vi "SwissSPAD Live_Save SS3 Data to HDF5_DVI.vi"(4 "Compression Level (0-9)":u8=9 max=9, 6 "Compression":bool, 7 "10-bit Gate Image":bool, 8 "error in (no error)":errorcluster, 9 "File Path::n":string="SS2 Live Gate Data Q", 10 "Gate Names":string[](array[string]), 11 "HDF5 ref":T1 format="%.0x") -> (0 "error out":errorcluster)   [LabVIEW 2021]
uses:
  <vilib>/addons/h5labview2/base/hid_t.ctl
  SwissSPAD Live_Settings List.ctl
  SwissSPAD Live_SS3 DAQ Parameters.ctl
  SwissSPAD Live_SS3 Gate Definition.ctl
  SS3 Gate Width Definition Mode.ctl
  SwissSPAD Live_Gate Type.ctl
  <vilib>/Utility/error.llb/DialogType.ctl
  <vilib>/addons/h5labview2/file/H5F.lvlib
  <vilib>/addons/h5labview2/group/H5G.lvlib
  Notebook/Notebook.lvlib
  Rich Text Box/Rich Text Box.lvlib
  Variant/Variant to Data/Variant to Data.lvlib
panel:
  out "File Path":string
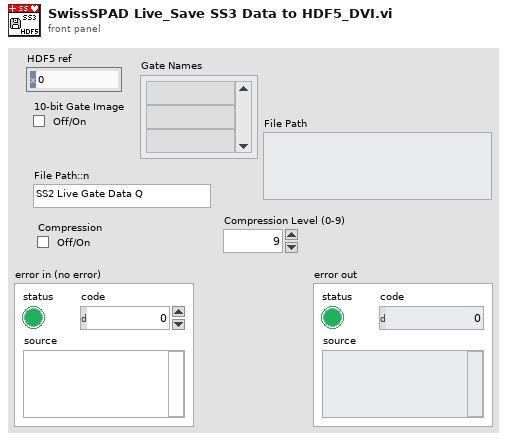
[diagram p1: front panel]
types:
  T1 = typedef "hid_t.ctl" = i32
  T2 = typedef "SwissSPAD Live_Settings List.ctl" = enum16{"FPGA:Bottom Half", "FPGA:Top Half", "FPGA:Bottom Bitfile Path", "FPGA:Top Bitfile Path", "FPGA:Bottom Bitstream Version", "FPGA:Top Bitstream Version", "FPGA:Auto Reset FPGA", "FPGA:Bottom FPGA Serial Number", "FPGA:Top FPGA Serial Number", "FPGA:Detector PCB Version", "Acquisition Parameters:Microlens", "Acquisition Parameters:SS2 DAQ Parameters", "Acquisition Parameters:Gate Configuration Array", "Acquisition Parameters:SS3 DAQ Parameters", "Acquisition Parameters:Buffer Size (# 8-bit Gates)", "File Information:File Information", "File Information:# Datasets in Series", "File Information:Scrambled File Flag", "File Information:SS3 Gate Slip Correction", "File Information:SS3 Hot Pixel Mismatch Detection", "File Information:Delay between Datasets", "File Information:Save Sum of All Gates Preview", "Image Parameters:Image ROI Information", "Image Parameters:Image Binning Options", "Image Parameters:SS3 Displayed Image", "Image Parameters:Image Display Options", "Image Parameters:Use Histogram Cursors", "Image Parameter:FPGA Data to Display", "UI Settings:Histogram Bins Number", "UI Settings:Histogram Bin Size", "UI Settings:Use Image Display Options", "UI Settings:Verbose Settings", "UI Settings:Verbose Saving"}
  T3 = typedef "SwissSPAD Live_Gate Type.ctl" = enum16{"INT", "G2"}
  T4 = typedef "SwissSPAD Live_SS3 DAQ Parameters.ctl" = cluster{"10 bits":bool, "# Exposure Sequences":u32, "# 1-bit Frame per Gate":u32, "Gate Shift":u32, "# Gate Pairs per Set":u32, "# Sets":u32, "Laser Period":dbl[unit], "Sync Period":dbl[unit], "Gate Offset":u32, "Auto-adjust Gate Offset":bool, "Gate Definition":T5, "Gate Width (ns)":dbl, "Reversed Shift":bool, "Intensity Mode":bool, "Gate Definition Mode":T6}
  T5 = typedef "SwissSPAD Live_SS3 Gate Definition.ctl" = cluster{"gs_psincdec_0":u32, "gs_psincdec_1":u32, "gs_no_shift_adj_1":u32, "gate_adj_2":u32}
  T6 = typedef "SS3 Gate Width Definition Mode.ctl" = enum32{"Item 0", "Item 1"}
  T7 = typedef "DialogType.ctl" = u16
  T8 = typedef "SwissSPAD Live_File Saving Task Information.ctl" = cluster{"File Path::n":string, "# Saved Images":i32, "# Images (Total)":i32, "File Size (Bytes)":i64}
  T9 = typedef "Rich Text Box.lvlib/Text Formatting.ctl" = cluster{"Font":string, "Text Color":T10, "Text Background Color":T10, "Text Style":enum16{"Regular", "Bold", "Italic", "Underline", "Strikeout"}, "Font Size (Points)":dbl, "Text Alignment":i32}
  T10 = typedef "Rich Text Box.lvlib/Text Colors.ctl" = enum16{"Unchanged", "Black", "Blue", "Brown", "Gray", "Green", "Orange", "Pink", "Red", "White"}
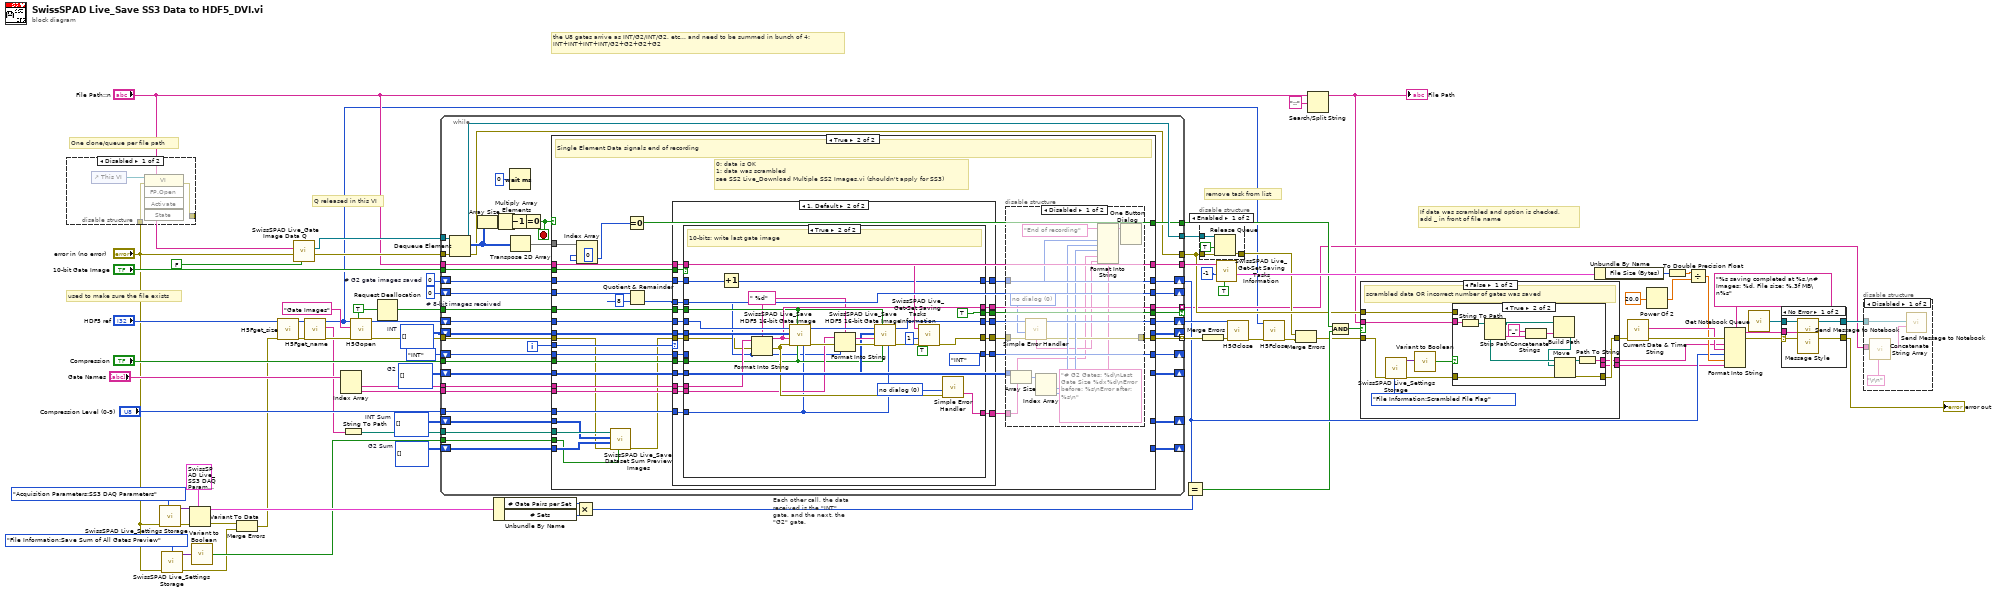
[diagram p0: block diagram]
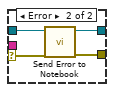
[diagram p5: hidden frame]
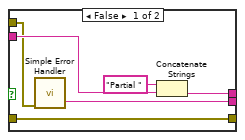
[diagram p6: hidden frame]
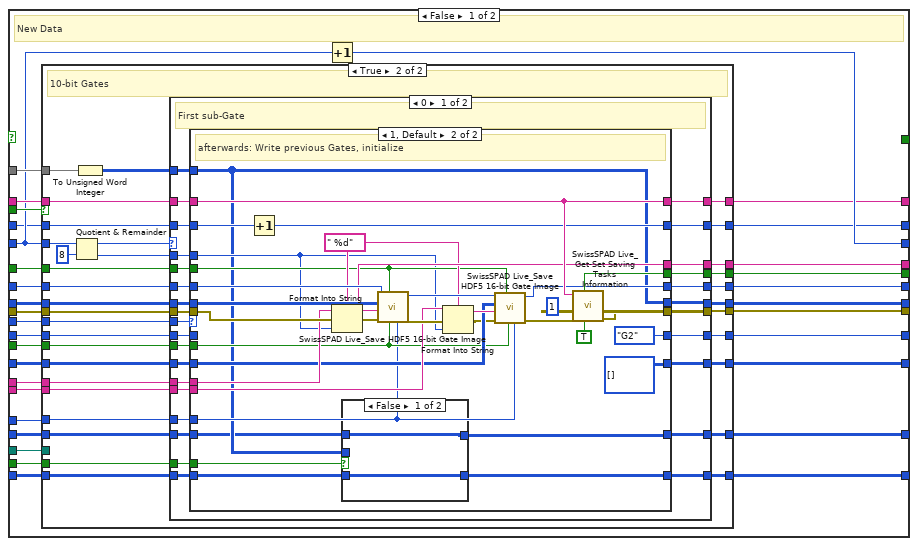
[diagram p8: hidden frame]
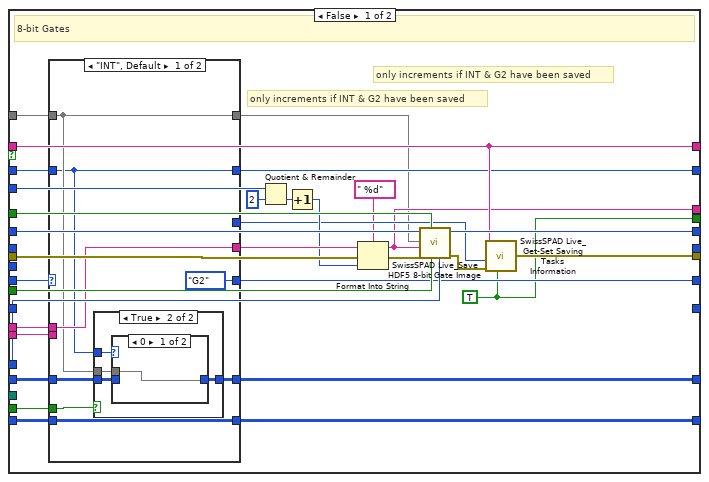
[diagram p9: hidden frame]
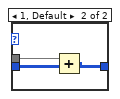
[diagram p11: hidden frame]
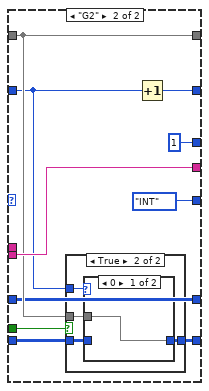
[diagram p12: hidden frame]
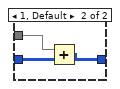
[diagram p14: hidden frame]
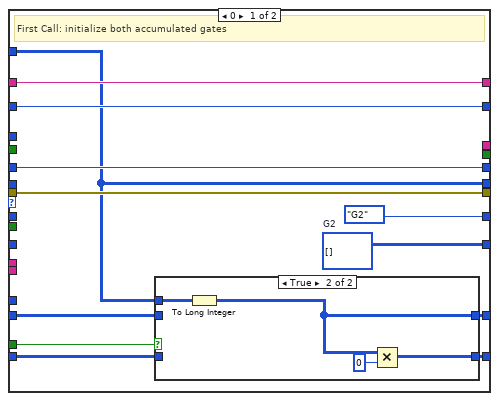
[diagram p15: hidden frame]
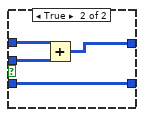
[diagram p17: hidden frame]
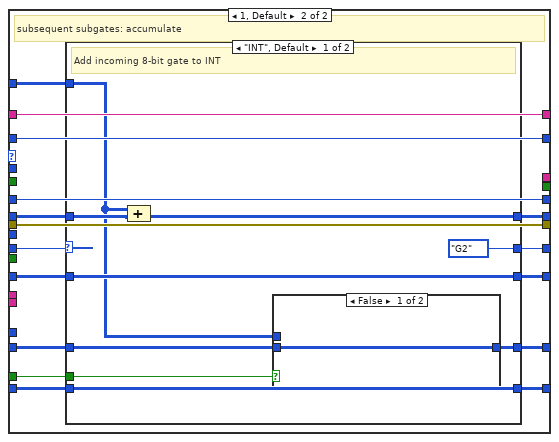
[diagram p18: hidden frame]
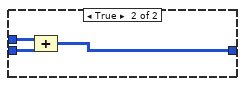
[diagram p19: hidden frame]
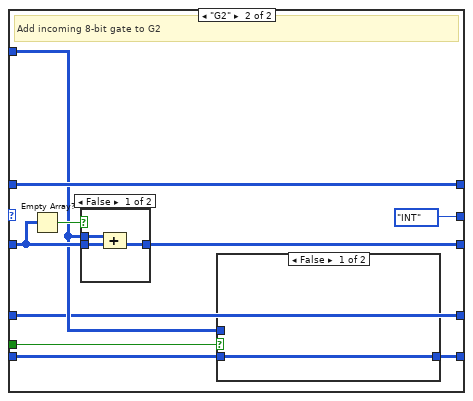
[diagram p20: hidden frame]
diagram:
  w11 = i32[][] []  # G2 Sum
  w12 = i32[][] []  # INT Sum
  w20 = u16[][] []  # G2
  w21 = u16[][] []  # INT
  w48 = 0  # # G2 gate images saved
  w57 = TRUE ("create? (F)")
  w78 = 0  # # 8-bit images received
  # "the U8 gates arrive as INT/G2/INT/G2, etc... and need to be summed in bunch of 4:\nINT+INT+INT+INT/G2+G2+G2+G2"
  # "remove task from list"
  # "Q released in this VI"
  # "If data was scrambled and option is checked,\nadd _ in front of file name"
  # "One clone/queue per file path"
  # "used to make sure the file exists"
  n1 = disable-structure shown="Disabled" {
    disable-tunnel: "error in (no error)" -> [w82 w83]
    disable-tunnel: [w81 w83] -> _
    frame Disabled {
      n2 = control-ref of="This VI"() -> (w80:refnum<vi>)
      n3 = invoke class="VI" method="FP.Open"(reference=w80, error in=w82) -> (error out=w81:errorcluster)  [unwired: 3 in, 4 out]
    }
    frame Enabled {
    }
  }
  n4 = call "SwissSPAD Live_Settings Storage.vi"("Settings List"=SwissSPAD_Live_Settings_List."Acquisition Parameters:SS3 DAQ Parameters", "Error In"="error in (no error)") -> ("Error Out"=w47:errorcluster, "Variant Data out"=w16:variant)  [unwired: 8 in]
  n5 = call "SwissSPAD Live_Settings Storage.vi"("Settings List"=SwissSPAD_Live_Settings_List."File Information:Save Sum of All Gates Preview", "Error In"="error in (no error)") -> ("Error Out"=w2:errorcluster, "Variant Data out"=w13:variant)  [unwired: 8 in]
  n6 = Variant To Data(error in=w47, type=T4 {"10 bits"=FALSE, "# Exposure Sequences"=0, "# 1-bit Frame per Gate"=0, "Gate Shift"=0, "# Gate Pairs per Set"=0, "# Sets"=1, "Laser Period"=0.0, "Sync Period"=0.0, "Gate Offset"=0, "Auto-adjust Gate Offset"=FALSE, "Gate Definition"={"gs_psincdec_0"=0, "gs_psincdec_1"=0, "gs_no_shift_adj_1"=0, "gate_adj_2"=0}, "Gate Width (ns)"=0.0, "Reversed Shift"=FALSE, "Intensity Mode"=FALSE, "Gate Definition Mode"=enum."Item 0"} ("SS3 DAQ Parameters"), Variant=w16) -> (data=w46:T4, error out=w4:errorcluster)
  n7 = call "Variant to Boolean.vi"("Variant"=w13) -> ("Value"=w10:bool)  [unwired: 8 in]
  n8 = Merge Errors(w4, w2) -> (w3:errorcluster)
  n9 = call <vilib>:"H5Fget_size.vi"("error in (no error)"=w3, "ref in"="HDF5 ref") -> ("error out"=w9:errorcluster, "ref out"=w8:T1)  [unwired: 7 in, 1 out]
  n10 = call "SwissSPAD Live_Gate Image Data Q.vi"("create if not found? (T)"=FALSE, "error in (no error)"="error in (no error)", "SwissSPAD Live Gate Image Data Q Name"="File Path::n") -> ("error out"=w30:errorcluster, "SwissSPAD Live Gate Image Data Q"=w29:refnum<queue>)  [unwired: 6 in, 1 out]
  n11 = call <vilib>:"H5Fget_name.vi"("error in (no error)"=w9, "ref in"=w8) -> ("error out"=w6:errorcluster, "name"=w5:string, "ref out"=w7:T1)  [unwired: 7 in]
  n12 = Index Array(array="Gate Names") -> (element #1=w23:string, element #2=w22:string)  [unwired: 2 in]
  n13 = String To Path(string=w5) -> (path=w1:path)
  n14 = call <vilib>:"H5Gopen.vi"("create? (F)"=w57, "error in (no error)"=w6, "name"="Gate Images", "ref in"=w7) -> ("error out"=w77:errorcluster, "group out"=w75:T1)  [unwired: 6 in]
  n15 = Request Deallocation(w57) -> ()
  n16 = while "Each other call, the data received is the \"INT\" gate, and the next, the \"G2\" gate." {
    tunnel: w29 -> [w126]
    tunnel: [w125] -> w79
    tunnel: w77 -> [w109]
    shift-right: [w116] -> _
    shift-left: w78 -> [w123]
    tunnel: w57 -> [w122]
    tunnel: [w121] -> w74 mode=indexing
    tunnel: "10-bit Gate Image" -> [w114]
    shift-right: [w112] -> _
    shift-left: w21 -> [w113]
    tunnel: [w84] -> w37
    tunnel: w30 -> [w108]
    tunnel: "File Path::n" -> [w107]
    tunnel: "Compression" -> [w106]
    tunnel: [w105] -> w53
    tunnel: [w103] -> w52
    tunnel: "Compression Level (0-9)" -> [w102]
    shift-right: [w100] -> w42
    shift-left: w48 -> [w101]
    shift-right: [w99] -> _
    shift-left: SwissSPAD_Live_Gate_Type."INT" -> [w98]
    tunnel: [w97] -> w31 mode=indexing if=w96
    tunnel: w23 -> [w94]
    tunnel: w22 -> [w95]
    shift-right: [w93] -> _
    shift-left: w20 -> [w92]
    shift-right: [w120] -> w73
    shift-left: w75 -> [w124]
    shift-right: [w88] -> _
    shift-left: w12 -> [w90]
    shift-right: [w86] -> _
    shift-left: w11 -> [w87]
    tunnel: w10 -> [w89]
    tunnel: w1 -> [w85]
    i -> [w111]
    stop <- w117 stop-if-true
    n17 = Dequeue Element(queue=w126, error in (no error)=w108) -> (queue out=w125:refnum<queue>, element=w115:u8[][], error out=w84:errorcluster)  [unwired: 1 in, 1 out]
    n18 = Array Size(array=w115) -> (size(s)=w118:i32[])
    n19 = Multiply Array Elements(1:w118) -> (0:w119:i32)
    n20 = Decrement(x=w119) -> (x-1=w104:i32)
    n21 = Wait (ms)(milliseconds to wait=u32 0) -> ()  [unwired: 1 out]
    n22 = Transpose 2D Array(2D array=w115) -> (transposed array=w110:u8[][])
    n23 = Equal To 0?(x=w104) -> (x = 0?=w117:bool)
    n24 = case shown="True" w117 {
      tunnel: w124 -> [w157 w425]
      tunnel: w109 -> [w154 w394]
      tunnel: w123 -> [w146 w404]
      tunnel: w122 -> [w158 w422]
      tunnel: [w148 w408] -> w121
      tunnel: [w156 w424] -> w120
      tunnel: [w155 w403] -> w116
      tunnel: w110 -> [w152 w419]
      tunnel: w114 -> [w153 w423]
      tunnel: w113 -> [w151 w426]
      tunnel: [w150 _] -> w112
      tunnel: w111 -> [w149 w420]
      tunnel: w107 -> [w147 w402]
      tunnel: w106 -> [w145 w421]
      tunnel: [w144 w402] -> w105
      tunnel: [_ w416] -> w103
      tunnel: w102 -> [w143 w415]
      tunnel: w101 -> [w142 w414]
      tunnel: [w141 w411] -> w100
      tunnel: [w133 w412] -> w99
      tunnel: w98 -> [w135 w413]
      tunnel: [w140 w407] -> w97
      tunnel: [w139 w406] -> w96
      tunnel: w95 -> [w138 w401]
      tunnel: w94 -> [w137 w400]
      tunnel: [w136 _] -> w93
      tunnel: w92 -> [w134 w399]
      tunnel: w90 -> [w132 w397]
      tunnel: w89 -> [w131 w393]
      tunnel: [w130 _] -> w88
      tunnel: w87 -> [w129 w396]
      tunnel: [w128 _] -> w86
      tunnel: w85 -> [w127 w398]
      frame False {
        # "New Data"
        n25 = case shown="True" w153 {
          tunnel: w158 -> [w186 w256]
          tunnel: [w184 w254] -> w148
          tunnel: w157 -> [w188 w258]
          tunnel: [w187 w257] -> w156
          tunnel: w154 -> [w190 w255]
          tunnel: w146 -> [w178 w245]
          tunnel: w152 -> [w164 w259]
          tunnel: w151 -> [_ w252]
          tunnel: [_ w250] -> w150
          tunnel: w149 -> [_ w253]
          tunnel: w147 -> [w182 w249]
          tunnel: w145 -> [w183 w244]
          tunnel: [w182 w243] -> w144
          tunnel: w143 -> [w181 w242]
          tunnel: w142 -> [w179 w241]
          tunnel: [w177 w240] -> w141
          tunnel: [w172 w239] -> w133
          tunnel: w135 -> [w180 w238]
          tunnel: [w169 w237] -> w140
          tunnel: [w168 w236] -> w139
          tunnel: w138 -> [w167 w234]
          tunnel: w137 -> [w166 w235]
          tunnel: [_ w233] -> w136
          tunnel: w134 -> [_ w232]
          tunnel: w132 -> [w165 w228]
          tunnel: w131 -> [w162 w231]
          tunnel: [w161 w230] -> w130
          tunnel: w129 -> [w160 w227]
          tunnel: [w159 w229] -> w128
          tunnel: w127 -> [_ _]
          frame False {
            w168 = TRUE ("Get (F)/Set")
            # "only increments if INT & G2 have been saved"
            # "only increments if INT & G2 have been saved"
            # "8-bit Gates"
            n26 = case shown="\"INT\", Default" w180 {
              tunnel: w179 -> [w191 w208]
              tunnel: [w191 w217] -> w177
              tunnel: [w197 w214] -> w176
              tunnel: [SwissSPAD_Live_Gate_Type."G2" SwissSPAD_Live_Gate_Type."INT"] -> w172
              tunnel: [_ 1 ("# New Images Saved")] -> w171
              tunnel: w167 -> [_ w214]
              tunnel: w166 -> [w197 _]
              tunnel: w165 -> [w195 w209]
              tunnel: w164 -> [w194 w211]
              tunnel: [w194 w211] -> w163
              tunnel: w162 -> [w196 w213]
              tunnel: [w193 w209] -> w161
              tunnel: w160 -> [w192 w212]
              tunnel: [w192 w210] -> w159
              frame "INT", Default {
                n27 = case shown="True" w196 {
                  tunnel: w195 -> [w199 w203]
                  tunnel: w194 -> [_ w202]
                  tunnel: [w199 w201] -> w193
                  tunnel: w191 -> [_ w200]
                  frame False {
                  }
                  frame True {
                    n28 = case shown="0" w200 {
                      tunnel: w203 -> [_ w207]
                      tunnel: w202 -> [w204 w206]
                      tunnel: [w204 w205] -> w201
                      frame 0 {
                      }
                      frame 1, Default {
                        n29 = Add(x=w206, y=w207) -> (x+y=w205:i32[][])
                      }
                    }
                  }
                }
              }
              frame "G2" {
                n30 = case shown="True" w213 {
                  tunnel: w211 -> [_ w222]
                  tunnel: w212 -> [w218 w221]
                  tunnel: [w218 w220] -> w210
                  tunnel: w208 -> [_ w219]
                  frame False {
                  }
                  frame True {
                    n31 = case shown="0" w219 {
                      tunnel: w222 -> [w223 w226]
                      tunnel: w221 -> [_ w225]
                      tunnel: [w223 w224] -> w220
                      frame 0 {
                      }
                      frame 1, Default {
                        n32 = Add(x=w226, y=w225) -> (x+y=w224:i32[][])
                      }
                    }
                  }
                }
                n33 = Increment(x=w208) -> (x+1=w217:i32)
              }
            }
            n34 = Quotient & Remainder(x=w178, y=2) -> (floor(x/y)=w174:i32)  [unwired: 1 out]
            n35 = Increment(x=w174) -> (x+1=w173:i32)
            n36 = Format Into String(format string=" %d", initial string=w176, error in=w190, w173) -> (resulting string=w169:string, error out=w189:errorcluster)
            n37 = call "SwissSPAD Live_Save HDF5 8-bit Gate Image.vi"("Compression Level (0-9)"=w181, "Compression"=w183, "Replace?"=w186, "error in (no error)"=w189, "Image Name"=w169, "Data"=w163, "ref in"=w188) -> ("error out"=w185:errorcluster, "ref out"=w187:T1)  [unwired: 3 in]
            n38 = call "SwissSPAD Live_Get-Set Saving Tasks Information.vi"("Get (F)/Set"=w168, "error in (no error)"=w185, "# New Images Saved (1)"=w171, "File Path::n"=w182) -> ("error out"=w184:errorcluster)  [unwired: 4 in, 3 out]
          }
          frame True {
            # "10-bit Gates"
            n39 = Quotient & Remainder(x=w245, y=8) -> (x-y*floor(x/y)=w246:i32, floor(x/y)=w247:i32)
            n40 = To Unsigned Word Integer(number=w259) -> (unsigned 16bit integer=w251:u16[][])
            n41 = case shown="0" w246 {
              tunnel: w258 -> [w288 w360]
              tunnel: [w287 w360] -> w257
              tunnel: w256 -> [w286 _]
              tunnel: w255 -> [w285 w361]
              tunnel: [w284 w361] -> w254
              tunnel: w253 -> [w283 _]
              tunnel: w247 -> [w282 _]
              tunnel: w252 -> [w280 w352]
              tunnel: w251 -> [w281 w359]
              tunnel: [w279 w358] -> w250
              tunnel: w249 -> [w278 w357]
              tunnel: w244 -> [w277 _]
              tunnel: [w276 w357] -> w243
              tunnel: w242 -> [w275 _]
              tunnel: w241 -> [w274 w356]
              tunnel: [w273 w356] -> w240
              tunnel: [w272 w351] -> w239
              tunnel: w238 -> [w271 w355]
              tunnel: [w270 _] -> w237
              tunnel: [w269 _] -> w236
              tunnel: w235 -> [w268 _]
              tunnel: w234 -> [w267 _]
              tunnel: [w266 w353] -> w233
              tunnel: w232 -> [w265 w354]
              tunnel: w231 -> [w264 w350]
              tunnel: [w263 w346] -> w230
              tunnel: [w262 w348] -> w229
              tunnel: w228 -> [w261 w347]
              tunnel: w227 -> [w260 w349]
              frame 0 {
                # "First sub-Gate"
                n42 = case shown="1, Default" w283 {
                  tunnel: w288 -> [w300 w339]
                  tunnel: [w300 w324] -> w287
                  tunnel: w286 -> [_ w315]
                  tunnel: w285 -> [w299 w332]
                  tunnel: [w299 w337] -> w284
                  tunnel: w282 -> [_ w313]
                  tunnel: w281 -> [w293 w311]
                  tunnel: [w293 w311] -> w279
                  tunnel: w280 -> [_ w338]
                  tunnel: w278 -> [w298 w336]
                  tunnel: w277 -> [_ w316]
                  tunnel: [w298 w336] -> w276
                  tunnel: w275 -> [_ w314]
                  tunnel: w274 -> [w297 w334]
                  tunnel: [w297 w333] -> w273
                  tunnel: [SwissSPAD_Live_Gate_Type."G2" SwissSPAD_Live_Gate_Type."G2"] -> w272
                  tunnel: w271 -> [_ _]
                  tunnel: [_ w329] -> w270
                  tunnel: [_ w328] -> w269
                  tunnel: w268 -> [_ w326]
                  tunnel: w267 -> [_ w321]
                  tunnel: [w296 u16[][] [] ("G2")] -> w266
                  tunnel: w265 -> [_ w319]
                  tunnel: w264 -> [w294 w312]
                  tunnel: [w292 w309] -> w263
                  tunnel: [w291 w307] -> w262
                  tunnel: w261 -> [w290 w310]
                  tunnel: w260 -> [w289 w308]
                  frame 0 {
                    w296 = u16[][] []  # G2
                    # "First Call: initialize both accumulated gates"
                    n43 = case shown="True" w294 {
                      tunnel: w293 -> [_ w306]
                      tunnel: [w302 w303] -> w292
                      tunnel: [w301 w305] -> w291
                      tunnel: w290 -> [w302 _]
                      tunnel: w289 -> [w301 _]
                      frame False {
                      }
                      frame True {
                        n44 = To Long Integer(number=w306) -> (32bit integer=w303:i32[][])
                        n45 = Multiply(x=w303, y=0) -> (x*y=w305:i32[][])
                      }
                    }
                  }
                  frame 1, Default {
                    w322 = " %d" ("format string")
                    w328 = TRUE ("Get (F)/Set")
                    # "afterwards: Write previous Gates, initialize"
                    n46 = Increment(x=w334) -> (x+1=w333:i32)
                    n47 = Format Into String(format string=w322, initial string=w326, error in=w332, w313) -> (resulting string=w329:string, error out=w331:errorcluster)
                    n48 = case shown="False" w312 {
                      tunnel: w311 -> [_ w344]
                      tunnel: w310 -> [w341 w345]
                      tunnel: [w341 w343] -> w309
                      tunnel: w308 -> [w340 w342]
                      tunnel: [w340 w342] -> w307
                      frame False {
                      }
                      frame True {
                        n49 = Add(x=w345, y=w344) -> (x+y=w343:i32[][])
                      }
                    }
                    n50 = call "SwissSPAD Live_Save HDF5 16-bit Gate Image.vi"("Compression Level (0-9)"=w314, "Compression"=w316, "Replace?"=w315, "error in (no error)"=w331, "Image Name"=w329, "Data"=w338, "ref in"=w339) -> ("error out"=w323:errorcluster, "ref out"=w325:T1)  [unwired: 3 in]
                    n51 = Format Into String(format string=w322, initial string=w321, error in=w323, w313) -> (resulting string=w320:string, error out=w318:errorcluster)
                    n52 = call "SwissSPAD Live_Save HDF5 16-bit Gate Image.vi"("Compression Level (0-9)"=w314, "Compression"=w316, "Replace?"=w315, "error in (no error)"=w318, "Image Name"=w320, "Data"=w319, "ref in"=w325) -> ("error out"=w317:errorcluster, "ref out"=w324:T1)  [unwired: 3 in]
                    n53 = call "SwissSPAD Live_Get-Set Saving Tasks Information.vi"("Get (F)/Set"=w328, "error in (no error)"=w317, "# New Images Saved (1)"=1 ("# New Images Saved"), "File Path::n"=w336) -> ("error out"=w337:errorcluster)  [unwired: 4 in, 3 out]
                  }
                }
              }
              frame 1, Default {
                # "subsequent subgates: accumulate"
                n54 = case shown="\"INT\", Default" w355 {
                  tunnel: w359 -> [w365 w378]
                  tunnel: [w368 w383] -> w358
                  tunnel: w354 -> [w370 w381]
                  tunnel: [w370 w384] -> w353
                  tunnel: w352 -> [w369 w383]
                  tunnel: [SwissSPAD_Live_Gate_Type."G2" SwissSPAD_Live_Gate_Type."INT"] -> w351
                  tunnel: w350 -> [w366 w379]
                  tunnel: w349 -> [w362 w377]
                  tunnel: [w362 w376] -> w348
                  tunnel: w347 -> [w364 w375]
                  tunnel: [w363 w375] -> w346
                  frame "INT", Default {
                    # "Add incoming 8-bit gate to INT"
                    n55 = Compound Arithmetic op=ADD(w365, w369) -> (w368:u16[][])
                    n56 = case shown="False" w366 {
                      tunnel: w365 -> [_ w373]
                      tunnel: w364 -> [w371 w374]
                      tunnel: [w371 w372] -> w363
                      frame False {
                      }
                      frame True {
                        n57 = Compound Arithmetic op=ADD(w373, w374) -> (w372:i32[][])
                      }
                    }
                  }
                  frame "G2" {
                    # "Add incoming 8-bit gate to G2"
                    n58 = Empty Array?(array=w381) -> (empty?=w380:bool)
                    n59 = case shown="False" w380 {
                      tunnel: w378 -> [w391 w392]
                      tunnel: [w390 w392] -> w384
                      tunnel: w381 -> [w389 _]
                      frame False {
                        n60 = Compound Arithmetic op=ADD(w391, w389) -> (w390:u16[][])
                      }
                      frame True {
                      }
                    }
                    n61 = case shown="False" w379 {
                      tunnel: w378 -> [_ w387]
                      tunnel: w377 -> [w385 w388]
                      tunnel: [w385 w386] -> w376
                      frame False {
                      }
                      frame True {
                        n62 = Compound Arithmetic op=ADD(w387, w388) -> (w386:i32[][])
                      }
                    }
                  }
                }
              }
            }
          }
        }
        n63 = Increment(x=w146) -> (x+1=w155:i32)
      }
      frame True {
        w418 = 0 ("index (row)")
        # "0: data is OK\n1: data was scrambled\nsee SS2 Live_Download Multiple SS2 Images.vi (shouldn't apply for SS3)"
        # "Single Element Data signals end of recording"
        n64 = Index Array(array=w419, index (row)=w418, index (col)=w418) -> (element=w417:u8)
        n65 = call "SwissSPAD Live_Save Dataset Sum Preview Images.vi"("Save Preview"=w393, "error in (no error)"=w394, "G2 Sum"=w396, "INT Sum"=w397, "HDF5 File Path"=w398) -> ("error out"=w395:errorcluster)  [unwired: 6 in]
        n66 = Equal To 0?(x=w417) -> (x = 0?=w416:bool)
        n67 = Quotient & Remainder(x=w404, y=8) -> (floor(x/y)=w403:i32)  [unwired: 1 out]
        n68 = case shown="1, Default" w420 {
          tunnel: w426 -> [_ w465]
          tunnel: w425 -> [w444 w464]
          tunnel: [w444 w463] -> w424
          tunnel: w395 -> [w443 w462]
          tunnel: w403 -> [_ w461]
          tunnel: [w443 w460] -> w409
          tunnel: w423 -> [_ w459]
          tunnel: w422 -> [_ w458]
          tunnel: w421 -> [_ w457]
          tunnel: w415 -> [_ w456]
          tunnel: w414 -> [w442 w455]
          tunnel: [w442 w454] -> w411
          tunnel: w413 -> [w441 w453]
          tunnel: [w441 w452] -> w412
          tunnel: [_ w451] -> w410
          tunnel: [_ w450] -> w407
          tunnel: [_ w449] -> w406
          tunnel: w402 -> [_ w448]
          tunnel: w401 -> [_ w447]
          tunnel: w400 -> [_ w446]
          tunnel: w399 -> [_ w445]
          frame 0 {
            # "no data ever received (FPGA timeout?)"
          }
          frame 1, Default {
            n69 = case shown="True" w459 {
              tunnel: w465 -> [_ w497]
              tunnel: w464 -> [w469 w498]
              tunnel: [w469 w482] -> w463
              tunnel: w462 -> [w468 w471]
              tunnel: [w468 w470] -> w460
              tunnel: w461 -> [_ w472]
              tunnel: w458 -> [_ w481]
              tunnel: w457 -> [_ w474]
              tunnel: w456 -> [_ w473]
              tunnel: w455 -> [w467 w491]
              tunnel: [w467 w486] -> w454
              tunnel: w453 -> [w466 _]
              tunnel: [w466 SwissSPAD_Live_Gate_Type."INT"] -> w452
              tunnel: [_ w494] -> w451
              tunnel: [_ w493] -> w450
              tunnel: [_ TRUE] -> w449
              tunnel: w448 -> [_ w487]
              tunnel: w447 -> [_ w479]
              tunnel: w446 -> [_ w478]
              tunnel: w445 -> [_ w475]
              frame False {
                # "8-bit data: nothing to do"
              }
              frame True {
                w495 = T7 0 items=["no dialog", "OK message", "continue or stop message", "OK message + warnings", "continue/stop + warnings"] ("type of dialog (OK msg:1)")
                w480 = " %d" ("format string")
                # "10-bits: write last gate image"
                n70 = Increment(x=w491) -> (x+1=w486:i32)
                n71 = Format Into String(format string=w480, initial string=w478, error in=w471, w472) -> (resulting string=w493:string, error out=w496:errorcluster)
                n72 = call "SwissSPAD Live_Save HDF5 16-bit Gate Image.vi"("Compression Level (0-9)"=w473, "Compression"=w474, "Replace?"=w481, "error in (no error)"=w496, "Image Name"=w493, "Data"=w497, "ref in"=w498) -> ("error out"=w485:errorcluster, "ref out"=w483:T1)  [unwired: 3 in]
                n73 = Format Into String(format string=w480, initial string=w479, error in=w485, w472) -> (resulting string=w476:string, error out=w484:errorcluster)
                n74 = call "SwissSPAD Live_Save HDF5 16-bit Gate Image.vi"("Compression Level (0-9)"=w473, "Compression"=w474, "Replace?"=w481, "error in (no error)"=w484, "Image Name"=w476, "Data"=w475, "ref in"=w483) -> ("error out"=w477:errorcluster, "ref out"=w482:T1)  [unwired: 3 in]
                n75 = call "SwissSPAD Live_Get-Set Saving Tasks Information.vi"("Get (F)/Set"=TRUE, "error in (no error)"=w477, "# New Images Saved (1)"=1 ("# New Images Saved"), "File Path::n"=w487) -> ("error out"=w470:errorcluster)  [unwired: 4 in, 3 out]
                n76 = call <vilib>:"Simple Error Handler.vi"("type of dialog (OK msg:1)"=w495, "error in (no error)"=w496) -> ("message"=w494:string)  [unwired: 3 in, 4 out]
              }
            }
          }
        }
        n77 = disable-structure shown="Disabled" {
          disable-tunnel: w411 -> [w437 _]
          disable-tunnel: w410 -> [w429 _]
          disable-tunnel: w409 -> [w434 w440]
          disable-tunnel: [w433 w440] -> w408
          disable-tunnel: w399 -> [w428 _]
          frame Disabled {
            w432 = T7 0 items=["no dialog", "OK message", "continue or stop message", "OK message + warnings", "continue/stop + warnings"] ("type of dialog (OK msg:1)")
            n78 = Array Size(array=w428) -> (size(s)=w427:i32[])
            n79 = call <vilib>:"Simple Error Handler.vi"("type of dialog (OK msg:1)"=w432, "error in (no error)"=w434) -> ("error out"=w433:errorcluster, "message"=w431:string)  [unwired: 3 in, 3 out]
            n80 = Index Array(array=w427) -> (element #1=w436:i32, element #2=w435:i32)  [unwired: 2 in]
            n81 = Format Into String(format string="# G2 Gates: %d\nLast Gate Size %dx%d\nError before: %s\nError after: %s\n" ("message"), initial string="End of recording" ("message"), w437, w436, w435, w429, w431) -> (resulting string=w438:string)  [unwired: 1 in, 1 out]
            n82 = One Button Dialog(message=w438) -> ()  [unwired: 1 in, 1 out]
          }
          frame Enabled {
          }
        }
      }
    }
  }
  n83 = Unbundle By Name(w46) -> ("# Gate Pairs per Set"=w44:u32, "# Sets"=w43:u32)
  n84 = Multiply(x=w44, y=w43) -> (x*y=w41:u32)
  n85 = Equal?(x=w42, y=w41) -> (x = y?=w39:bool)
  n86 = disable-structure shown="Enabled" {
    disable-tunnel: w79 -> [w502 _]
    disable-tunnel: w37 -> [w501 w503]
    disable-tunnel: [w500 w503] -> w36
    frame Enabled {
      n87 = Release Queue(queue=w502, force destroy? (F)=TRUE, error in (no error)=w501) -> (error out=w500:errorcluster)  [unwired: 2 out]
    }
    frame Disabled {
    }
  }
  n88 = Merge Errors(w74) -> (w71:errorcluster)
  n89 = call "SwissSPAD Live_Get-Set Saving Tasks Information.vi"("Get (F)/Set"=TRUE, "# New Images Saved (1)"=-1 ("# New Images Saved"), "File Path::n"=w53) -> ("Complete Saving Task Information"=w54:T8)  [unwired: 5 in, 3 out]
  n90 = call <vilib>:"H5Gclose.vi"("error in (no error)"=w71, "group in"=w73) -> ("error out"=w72:errorcluster)  [unwired: 9 in]
  n91 = call <vilib>:"H5Fclose.vi"("error in (no error)"=w72, "ref"=w7) -> ("error out"=w35:errorcluster)  [unwired: 9 in]
  n92 = Merge Errors(w36, w35) -> (w34:errorcluster)
  n93 = Search/Split String(string="File Path::n", search string/char (-)="::") -> (substring before match=w25:string)  [unwired: 1 in, 2 out]
  "File Path" <- w25
  n94 = Compound Arithmetic op=AND(w52, w39) -> (w40:bool)
  n95 = case shown="False" w40 {
    tunnel: w34 -> [w513 w531]
    tunnel: [w509 w531] -> w51
    tunnel: w25 -> [w512 w532]
    tunnel: [w508 w532] -> w50
    tunnel: w37 -> [w507 _]
    tunnel: [w506 _] -> w38
    frame False {
      # "scrambled data OR incorrect number of gates was saved"
      n96 = call "SwissSPAD Live_Settings Storage.vi"("Settings List"=SwissSPAD_Live_Settings_List."File Information:Scrambled File Flag", "Error In"=w513) -> ("Error Out"=w510:errorcluster, "Variant Data out"=w504:variant)  [unwired: 8 in]
      n97 = call "Variant to Boolean.vi"("Variant"=w504) -> ("Value"=w511:bool)  [unwired: 8 in]
      n98 = case shown="True" w511 {
        tunnel: w512 -> [w518 w530]
        tunnel: w510 -> [w519 w527]
        tunnel: [w519 w521] -> w509
        tunnel: [w517 w520] -> w508
        tunnel: w507 -> [w515 _]
        tunnel: [w514 _] -> w506
        frame False {
          n99 = call <vilib>:"Simple Error Handler.vi"("error in (no error)"=w515) -> ("message"=w514:string)  [unwired: 4 in, 4 out]
          n100 = Concatenate Strings("Partial " ("string"), w518) -> (w517:string)
        }
        frame True {
          n101 = String To Path(string=w530) -> (path=w526:path)
          n102 = Strip Path(path=w526) -> (stripped path=w525:path, name=w529:string)
          n103 = Concatenate Strings("_" ("string"), w529) -> (w524:string)
          n104 = Build Path(base path=w525, name or relative path=w524) -> (appended path=w523:path)
          n105 = Move(source path=w526, error in=w527, 10:w523) -> (error out=w521:errorcluster, 3:w522:path)  [unwired: 2 in, 1 out]
          n106 = Path To String(path=w522) -> (string=w520:string)
        }
      }
    }
    frame True {
      # "Data is not scrambled AND correct number of gates was saved"
    }
  }
  n107 = Unbundle By Name(w54) -> ("File Size (Bytes)"=w63:i64)
  n108 = call "Current Date & Time String.vi"("Error In"=w51) -> ("Error Out"=w65:errorcluster, "time string"=w64:string)  [unwired: 8 in, 1 out]
  n109 = Power Of 2(x=20.0) -> (2^x=w61:dbl)
  n110 = To Double Precision Float(number=w63) -> (double precision float=w59:dbl)
  n111 = Divide(x=w59, y=w61) -> (x/y=w60:dbl)
  n112 = Format Into String(format string="%s saving completed at %s.\n# Images: %d, File size: %.3f MB\n%s", error in=w65, w50, w64, w42, w60, w38) -> (resulting string=w67:string, error out=w68:errorcluster)  [unwired: 1 in]
  n113 = call "Get Notebook Queue.vi"() -> ("Notebook Queue"=w69:refnum<queue>)  [unwired: 9 in]
  n114 = case shown="No Error" w68 {
    selector: w68 -> [w536 w540]
    tunnel: w69 -> [w533 w538]
    tunnel: w67 -> [w535 _]
    tunnel: [w534 w539] -> w33
    tunnel: [w533 w538] -> w32
    frame No Error {
      n115 = call "Message Style.vi"() -> ("Message Formatting"=w537:T9)
      n116 = call "Send Message to Notebook.vi"("Text Formatting"=w537, "Error In"=w536, "Message"=w535, "Notebook Queue"=w533) -> ("Error Out"=w534:errorcluster)  [unwired: 4 in, 1 out]
    }
    frame Error {
      n117 = call "Send Error to Notebook.vi"("error in (no error)"=w540, "Notebook Q"=w538) -> ("Error Out"=w539:errorcluster)  [unwired: 9 in]
    }
  }
  "error out" <- w33
  n118 = disable-structure shown="Disabled" {
    disable-tunnel: w32 -> [w544 _]
    disable-tunnel: w31 -> [w541 _]
    frame Disabled {
      n119 = call "Concatenate String Array.vi"("Separator (TAB)"="\r\n", "String Array"=w541) -> ("Formatted String"=w543:string)  [unwired: 9 in]
      n120 = call "Send Message to Notebook.vi"("Message"=w543, "Notebook Queue"=w544) -> ()  [unwired: 9 in, 1 out]
    }
    frame Enabled {
    }
  }
